vi "DigitalOutDividerSet.vi"(7 "divinit":u32, 8 "error in (no error)":errorcluster caption="错误输入（无错误）", 9 "div":u32=1, 10 "ch":i32, 11 "handle":u64) -> (0 "error out":errorcluster caption="错误输出", 1 "Frequency(Hz)":i32=9600, 2 "function return":i32, 3 "handle out":u64)   [LabVIEW 2018]
doc: "Set pos. or neg. Supply voltage"
uses:
  InstrumentsPlayground.lvlib
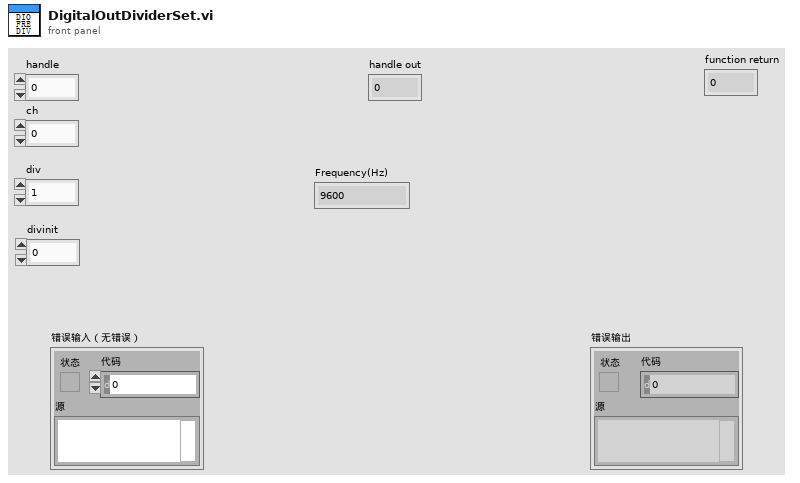
[diagram p1: front panel]
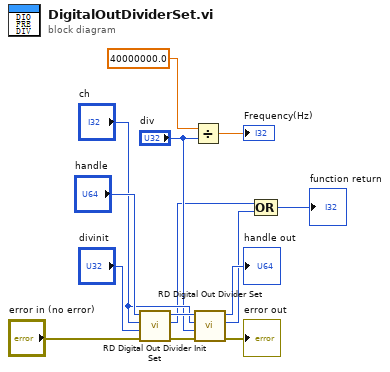
[diagram p0: block diagram]
diagram:
  n1 = call "RD Digital Out Divider Init Set.vi"("error in (no error)"="error in (no error)", "divinit"="divinit", "ch"="ch", "handle"="handle") -> ("error out"=w12:errorcluster, "function return"=w1:i32, "handle out"=w10:u64)  [unwired: 5 in]
  n2 = Divide(x=40000000.0, y="div") -> (x/y=→"Frequency(Hz)":dbl)
  n3 = call "RD Digital Out Divider Set.vi"("error in (no error)"=w12, "div"="div", "ch"="ch", "handle"=w10) -> ("error out"=→"error out":errorcluster, "function return"=w3:i32, "handle out"=→"handle out":u64)  [unwired: 5 in]
  n4 = Compound Arithmetic op=OR(w1, w3) -> (→"function return":i32)
